vi "Request Data JSON.vi"(8 "error in (no error)":errorcluster, 11 "SetProfileParameter in":refnum<class "SetProfileParameter.lvclass">) -> (0 "error out":errorcluster, 2 "Request Data JSON":string, 3 "SetProfileParameter out":refnum<class "SetProfileParameter.lvclass">)   [LabVIEW 2022 SP3, in "obs-websocket-lv.lvlib" / "SetProfileParameter.lvclass"]
uses:
  SetProfileParameter.lvclass
  SetProfileParameter.lvclass/SetProfileParameter.ctl
  <vilib>/IlluminatedG/lv-web-crypto/lv-json/JSON/JSON.lvlib
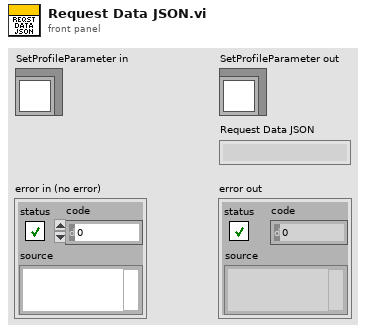
[diagram p1: front panel]
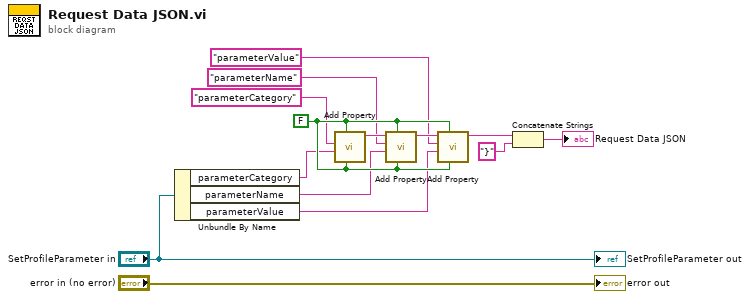
[diagram p0: block diagram]
diagram:
  w7 = FALSE ("Include Empty?")
  n1 = Unbundle By Name("SetProfileParameter in") -> ("parameterCategory"=w3:string, "parameterName"=w2:string, "parameterValue"=w1:string)
  n2 = call <vilib>:"Add Property.vi"("String?"=w7, "Include Empty?"=w7, "Value"=w3, "Property Name"="parameterCategory") -> ("String out"=w12:string)  [unwired: 7 in]
  n3 = call <vilib>:"Add Property.vi"("String?"=w7, "Include Empty?"=w7, "Value"=w2, "Property Name"="parameterName", "String In"=w12) -> ("String out"=w11:string)  [unwired: 6 in]
  n4 = call <vilib>:"Add Property.vi"("String?"=w7, "Include Empty?"=w7, "Value"=w1, "Property Name"="parameterValue", "String In"=w11) -> ("String out"=w10:string)  [unwired: 6 in]
  n5 = Concatenate Strings(w10, "}" ("string")) -> (→"Request Data JSON":string)
  "error out" <- "error in (no error)"
  "SetProfileParameter out" <- "SetProfileParameter in"
